vi "DrawImageLowLevel.vi"(0 "Image":T2 {"Dialogs" format="%.0b"}, 1 "Position":cluster{"left":i16, "top":i16}, 2 "Color Table":T1(ring), 3 "Autoscale?":bool, 4 "picture in":picture) -> (5 "new picture":picture, 6 "dimensions":cluster{"Width":i32, "Height":i32})   [LabVIEW 2024]
uses:
  <userlib>/ImageProcessing/QTLIB_2595_LV86/QT_Image.ctl
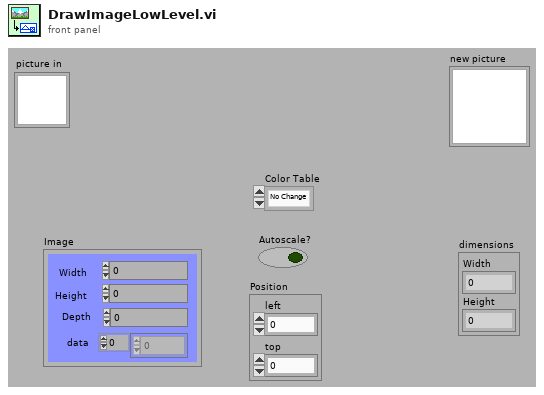
[diagram p1: front panel]
types:
  T1 = enum16{"No Change", "Apricot", "Carnation", "Ether", "Greyscale", "Greyscale-banded", "Hot Metal", "Lava Waves", "Mac", "Morning Glory", "Rainbow", "Rainbow-banded", "Rainbow-inverted", "Rainbow-striped", "Saturn", "Seismic", "Space"}
  T2 = typedef "QT_Image.ctl" = cluster{"Width":i32, "Height":i32, "Depth":i32, "data":u8[], "Compressed data":u8[], "Color table":u32[], "Duration":i32, "Options":i32, "Timestamp":i32, "ID":i32, "Reserved":i32, "Dialogs":u32}
  T3 = cluster{"left":i16, "top":i16, "right":i16, "bottom":i16}
  T4 = enum16{"Apricot", "Carnation", "Ether", "Greyscale", "Greyscale-banded", "Hot Metal", "Lava Waves", "Mac", "Morning Glory", "Rainbow", "Rainbow-banded", "Rainbow-inverted", "Rainbow-striped", "Saturn", "Seismic", "Space"}
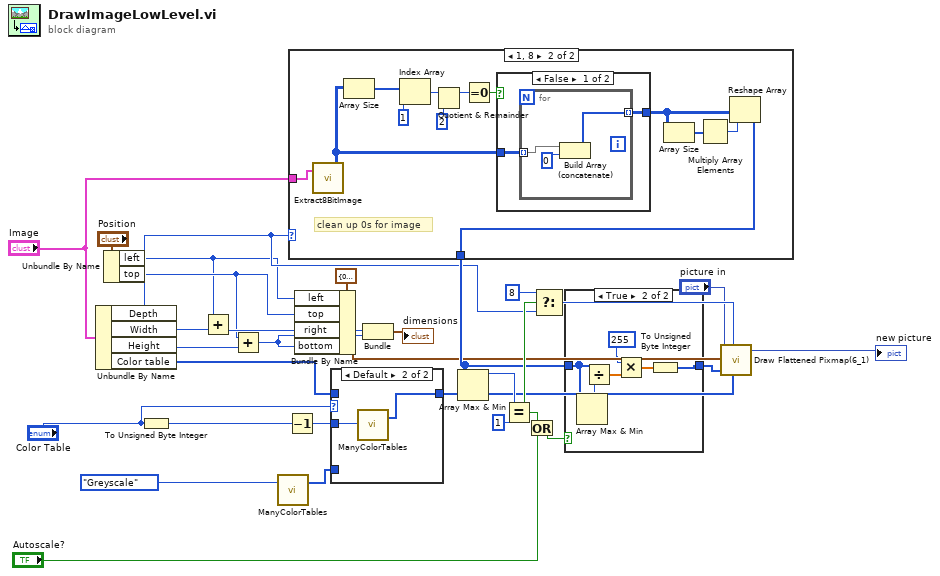
[diagram p0: block diagram]
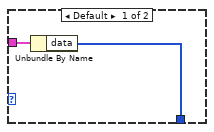
[diagram p2: hidden frame]
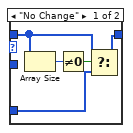
[diagram p5: hidden frame]
diagram:
  n1 = Unbundle By Name("Image") -> ("Depth"=w5:i32, "Width"=w3:i32, "Height"=w6:i32, "Color table"=w18:u32[])
  n2 = Unbundle By Name("Position") -> ("left"=w1:i16, "top"=w2:i16)
  n3 = To Unsigned Byte Integer(number="Color Table") -> (unsigned 8bit integer=w15:u8)
  n4 = Add(x=w1, y=w3) -> (x+y=w8:i32)
  n5 = Add(x=w2, y=w6) -> (x+y=w7:i32)
  n6 = call <userlib>:"ManyColorTables.vi"("Color Table"=T4."Greyscale") -> ("Color Table Out"=w25:u32[])  [unwired: 2 out]
  n7 = Decrement(x=w15) -> (x-1=w16:u8)
  n8 = case shown="1, 8" w5 {
    tunnel: "Image" -> [w32 w42]
    tunnel: [w31 w41] -> w26
    frame Default {
      n9 = Unbundle By Name(w32) -> ("data"=w31:u8[])
    }
    frame 1, 8 {
      # "clean up 0s for image"
      n10 = call <userlib>:"Extract8BitImage.vi"("Image in"=w42) -> ("Intensity Graph"=w33:u8[][])  [unwired: 1 in, 1 out]
      n11 = Array Size(array=w33) -> (size(s)=w35:i32[])
      n12 = Index Array(array=w35, index=1) -> (element=w38:i32)
      n13 = Quotient & Remainder(x=w38, y=2) -> (x-y*floor(x/y)=w39:i32)  [unwired: 1 out]
      n14 = Equal To 0?(x=w39) -> (x = 0?=w36:bool)
      n15 = case shown="False" w36 {
        tunnel: [w46 w50] -> w34
        tunnel: w33 -> [w45 w50]
        frame False {
          n16 = for {
            tunnel: [w48] -> w46 mode=indexing
            tunnel: w45 -> [w47] mode=indexing
            n17 = Build Array (concatenate)(w47, u8 0) -> (w48:u8[])
          }
        }
        frame True {
        }
      }
      n18 = Array Size(array=w34) -> (size(s)=w43:i32[])
      n19 = Multiply Array Elements(1:w43) -> (0:w44:i32)
      n20 = Reshape Array(w34, w44) -> (w41:u8[])
    }
  }
  n21 = Bundle By Name(cluster=T3 {"left"=0, "top"=0, "right"=0, "bottom"=0} ("rect"), "left"=w1, "top"=w2, "right"=w8, "bottom"=w7) -> (w13:T3)
  n22 = case shown="Default" "Color Table" {
    tunnel: w16 -> [_ w57]
    tunnel: [w51 w56] -> w17
    tunnel: w18 -> [w53 _]
    tunnel: w25 -> [w52 _]
    frame "No Change" {
      n23 = Array Size(array=w53) -> (size(s)=w55:i32)
      n24 = Not Equal To 0?(x=w55) -> (x != 0?=w54:bool)
      n25 = Select(t=w53, s=w54, f=w52) -> (s? t:f=w51:u32[])
    }
    frame Default {
      n26 = call <userlib>:"ManyColorTables.vi"("Color Table"=w57) -> ("Color Table Out"=w56:u32[])  [unwired: 2 out]
    }
  }
  n27 = Bundle(w8, w7) -> (→"dimensions":cluster{i32, i32})  [unwired: 1 out]
  n28 = Array Max & Min(array=w26) -> (max value=w27:u8)  [unwired: 3 out]
  n29 = Equal?(x=w27, y=u8 1) -> (x = y?=w28:bool)
  n30 = Or(x=w28, y="Autoscale?") -> (x .or. y?=w23:bool)
  n31 = Select(t=8, s=w28, f=w5) -> (s? t:f=w29:i32)
  n32 = case shown="True" w23 {
    tunnel: [w58 w59] -> w19
    tunnel: w26 -> [w58 w64]
    frame False {
    }
    frame True {
      n33 = Array Max & Min(array=w64) -> (max value=w63:u8)  [unwired: 3 out]
      n34 = Divide(x=w64, y=w63) -> (x/y=w62:dbl[])
      n35 = Multiply(x=i16 255 ("left"), y=w62) -> (x*y=w60:dbl[])
      n36 = To Unsigned Byte Integer(number=w60) -> (unsigned 8bit integer=w59:u8[])
    }
  }
  n37 = call <vilib>:"Draw Flattened Pixmap(6_1).vi"("picture"="picture in", "bit depth(8)"=w29, "rect"=w13, "flattened pixmap data"=w19, "color table"=w17) -> ("new picture"=→"new picture":picture)  [unwired: 4 out]
